vi "DTbl Digital to Binary U32.vi"(8 "error in (no error)":errorcluster, 11 "digital data":digitaldata) -> (0 "error out":errorcluster, 3 "binary array":u32[](array[numeric]))   [LabVIEW 2020]
doc: "Converts a digital waveform or set of digital data to a binary array of unsigned integers. You must manually select the polymorphic instance you want to use."
uses:
  DTbl Digital Size.vi
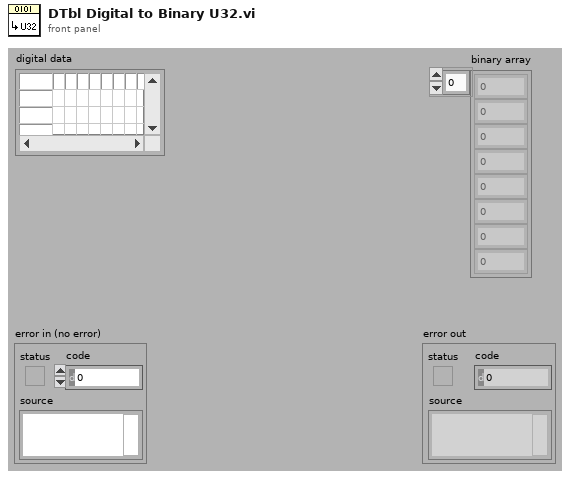
[diagram p1: front panel]
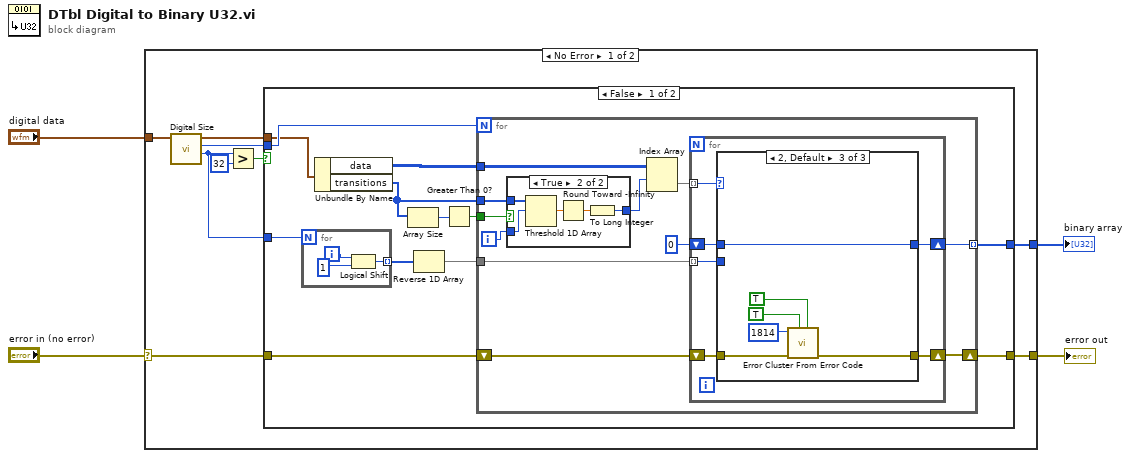
[diagram p0: block diagram]
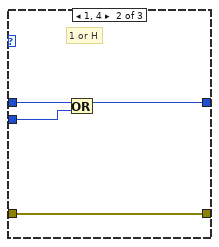
[diagram p3: hidden frame]
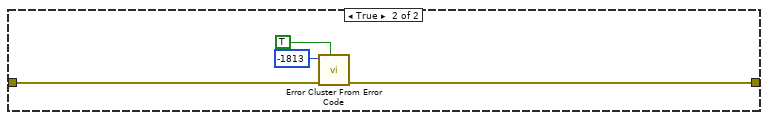
[diagram p5: hidden frame]
diagram:
  n1 = case shown="No Error" "error in (no error)" {
    selector: "error in (no error)" -> [w10 w68]
    tunnel: [w9 w68] -> w3
    tunnel: "digital data" -> [w13 _]
    tunnel: [w6 _] -> w1
    frame No Error {
      n2 = call-poly "Digital Size.vi"("digital data in"=w13) -> ("number of signals"=w5:i32, "number of samples"=w7:i32, "digital data out"=w8:digitaldata)  [unwired: 7 in, 1 out]
      n3 = Greater?(x=w5, y=32) -> (0:w11:bool)
      n4 = case shown="False" w11 {
        tunnel: w10 -> [w25 w67]
        tunnel: [w24 w66] -> w9
        tunnel: w8 -> [w22 _]
        tunnel: w7 -> [w23 _]
        tunnel: [w15 _] -> w6
        tunnel: w5 -> [w14 _]
        frame False {
          n5 = for {
            N: w14 -> [_]
            tunnel: [w26] -> w17 mode=indexing
            i -> [w27]
            n6 = Logical Shift(y=w27, x=u32 1) -> (x << y=w26:u32)
          }
          n7 = Unbundle By Name(w22) -> ("data"=w20:u8[][], "transitions"=w19:u32[])
          n8 = Array Size(array=w19) -> (size(s)=w21:i32)
          n9 = Reverse 1D Array(array=w17) -> (reversed array=w16:u32[])
          n10 = Greater Than 0?(x=w21) -> (x > 0?=w18:bool)
          n11 = for {
            N: w23 -> [_]
            shift-right: [w30] -> w24
            shift-left: w25 -> [w31]
            tunnel: w20 -> [w36]
            tunnel: w19 -> [w38]
            tunnel: w18 -> [w39]
            tunnel: w16 -> [w33]
            tunnel: [w29] -> w15 mode=indexing
            i -> [w37]
            n12 = case shown="True" w39 {
              tunnel: w38 -> [_ w63]
              tunnel: w37 -> [w58 w62]
              tunnel: [w58 w59] -> w35
              frame False {
              }
              frame True {
                n13 = Threshold 1D Array(2:w62, 3:w63) -> (0:w61:dbl)  [unwired: 1 in]
                n14 = Round Toward -Infinity(1:w61) -> (0:w60:dbl)
                n15 = To Long Integer(number=w60) -> (32bit integer=w59:i32)
              }
            }
            n16 = Index Array(array=w36, index (row)=w35) -> (element=w34:u8[])  [unwired: 1 in]
            n17 = for {
              tunnel: w34 -> [w45] mode=indexing
              tunnel: w33 -> [w42] mode=indexing
              shift-right: [w43] -> w29
              shift-left: u32 0 -> [w44]
              shift-right: [w40] -> w30
              shift-left: w31 -> [w41]
              n18 = case shown="2, Default" w45 {
                tunnel: w44 -> [w47 w51 w57]
                tunnel: [w47 w49 w57] -> w43
                tunnel: w42 -> [_ w50 _]
                tunnel: w41 -> [w46 w48 w56]
                tunnel: [w46 w48 w53] -> w40
                frame 0, 3 {
                  # "0 or L"
                }
                frame 1, 4 {
                  # "1 or H"
                  n19 = Or(x=w51, y=w50) -> (x .or. y?=w49:u32)
                }
                frame 2, Default {
                  n20 = call "Error Cluster From Error Code.vi"("is warning? (False)"=TRUE, "show call chain? (False)"=TRUE, "error in (no error)"=w56, "error code (0)"=1814) -> ("error out"=w53:errorcluster)  [unwired: 5 in]
                }
              }
            }
          }
        }
        frame True {
          n21 = call "Error Cluster From Error Code.vi"("show call chain? (False)"=TRUE, "error in (no error)"=w67, "error code (0)"=-1813) -> ("error out"=w66:errorcluster)  [unwired: 6 in]
        }
      }
    }
    frame Error {
    }
  }
  "binary array" <- w1
  "error out" <- w3
